vi "New Parameter Message.vi"(8 "error in (no error)":errorcluster, 10 "New parameter":variant, 11 "Syringe Pump in":refnum<class "Syringe Pump.lvclass">) -> (0 "error out":errorcluster, 2 "New Parameter Message":T1, 3 "Syringe Pump out":refnum<class "Syringe Pump.lvclass">)   [LabVIEW 2020, in "RxnRover.lvlib" / "Syringe Pump.lvclass"]
doc: "Dynamic dispatch for each child controller type to provide it's proper message for setting a new parameter value (setpoint)."
uses:
  Syringe Pump.lvclass
  <userlib>/RxnRover/DynamicReentrant/src/Type Defs/Message.ctl
  Syringe Pump.lvclass/Syringe Pump.ctl
  <userlib>/RxnRover/DynamicReentrant/Dynamic Reentrant.lvlib
  RxnRover.lvlib
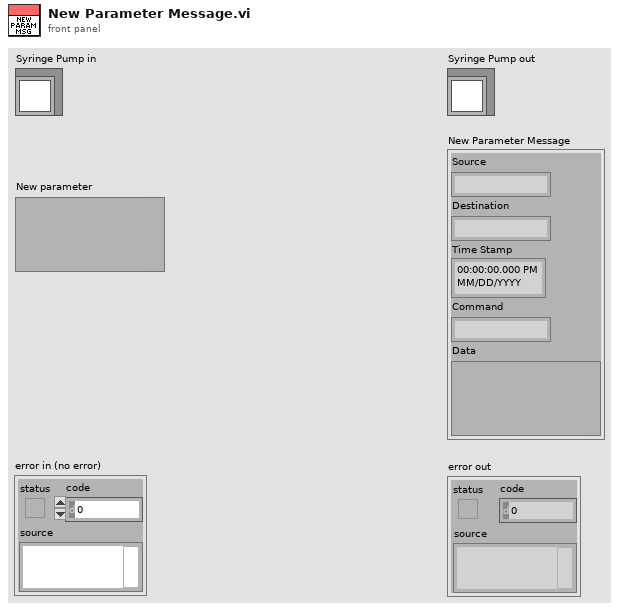
[diagram p1: front panel]
types:
  T1 = typedef "Dynamic Reentrant.lvlib/Message.ctl" = cluster{"Source":string, "Destination":string, "Time Stamp":timestamp, "Command":string, "Data":variant}
  T2 = typedef "RxnRover.lvlib/Supported Parameter Variant Types.ctl" = enum16{"Unsupported", "Numeric", "Boolean", "String", "Path"}
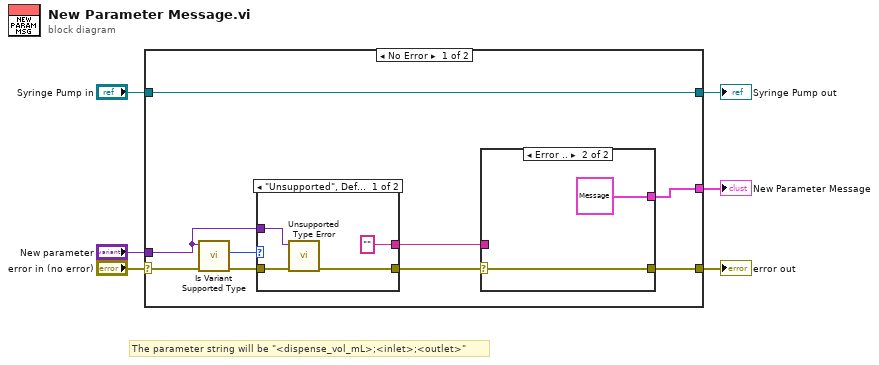
[diagram p0: block diagram]
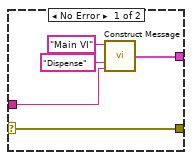
[diagram p2: hidden frame]
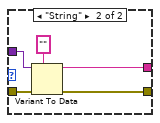
[diagram p3: hidden frame]
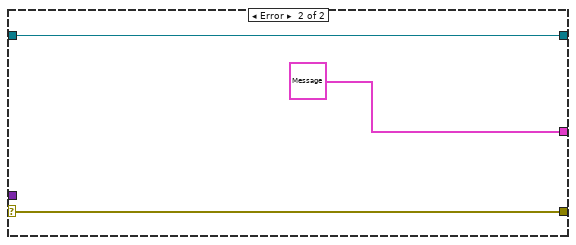
[diagram p4: hidden frame]
diagram:
  # "The parameter string will be \"<dispense_vol_mL>;<inlet>;<outlet>\""
  n1 = case shown="No Error" "error in (no error)" {
    selector: "error in (no error)" -> [w11 w33]
    tunnel: "New parameter" -> [w10 _]
    tunnel: [w14 T1 {"Source"="", "Destination"="", "Time Stamp"=timestamp(0 s since 1904-01-01), "Command"="", "Data"=variant} ("output cluster")] -> w5
    tunnel: [w7 w33] -> w6
    tunnel: "Syringe Pump in" -> [w15 w32]
    tunnel: [w15 w32] -> w4
    frame No Error {
      n2 = call "Is Variant Supported Type.vi"("error in (no error)"=w11, "variant"=w10) -> ("error out"=w13:errorcluster, "Type"=w12:T2)  [unwired: 7 in, 1 out]
      n3 = case shown="\"Unsupported\", Default" w12 {
        tunnel: w10 -> [w25 w28]
        tunnel: ["" w27] -> w8
        tunnel: [w26 w30] -> w9
        tunnel: w13 -> [w24 w31]
        frame "Unsupported", Default {
          n4 = call "Unsupported Type Error.vi"("error in (no error)"=w24, "Variant"=w25) -> ("Unsupported Parameter Variant Type"=w26:errorcluster)  [unwired: 9 in]
        }
        frame "String" {
          n5 = Variant To Data(error in=w31, type="", Variant=w28) -> (data=w27:string, error out=w30:errorcluster)
        }
      }
      n6 = case shown="Error .." w9 {
        selector: w9 -> [w16 w22]
        tunnel: [w18 T1 {"Source"="", "Destination"="", "Time Stamp"=timestamp(0 s since 1904-01-01), "Command"="", "Data"=variant} ("Message Cluster")] -> w14
        tunnel: w8 -> [w17 _]
        tunnel: [w16 w22] -> w7
        frame No Error {
          n7 = call <userlib>:"Construct Message.vi"("Data"=w17, "Command"="Dispense", "Source"="Main VI") -> ("Message Cluster"=w18:T1)  [unwired: 3 in]
        }
        frame Error {
        }
      }
    }
    frame Error {
    }
  }
  "error out" <- w6
  "Syringe Pump out" <- w4
  "New Parameter Message" <- w5
